vi "Error Cluster From Error Code_subroutine.vi"(4 "is warning? (False)":bool, 5 "show call chain? (False)":bool, 6 "error in (no error)":errorcluster, 8 "error message (\"\")":string, 9 "error code (0)":i32) -> (0 "error out":errorcluster)   [LabVIEW 2019, in "Tools.lvlib"]
doc: "Converts an error or warning code to an error cluster. This VI is useful when you receive a return value from a shared library call or when you return user-defined error codes."
uses:
  <vilib>/Utility/error.llb/whitespace.ctl
  Tools.lvlib
panel:
  in  "call chain header":string="\n<b>Complete call chain:</b>"
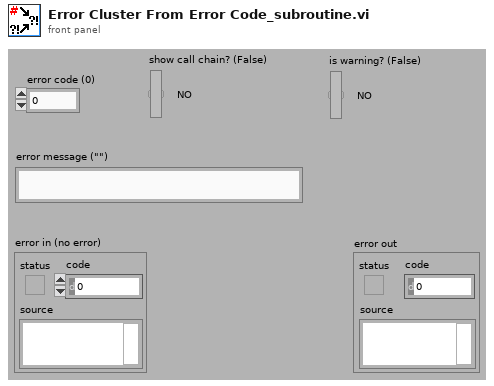
[diagram p1: front panel]
types:
  T1 = typedef "whitespace.ctl" = u16
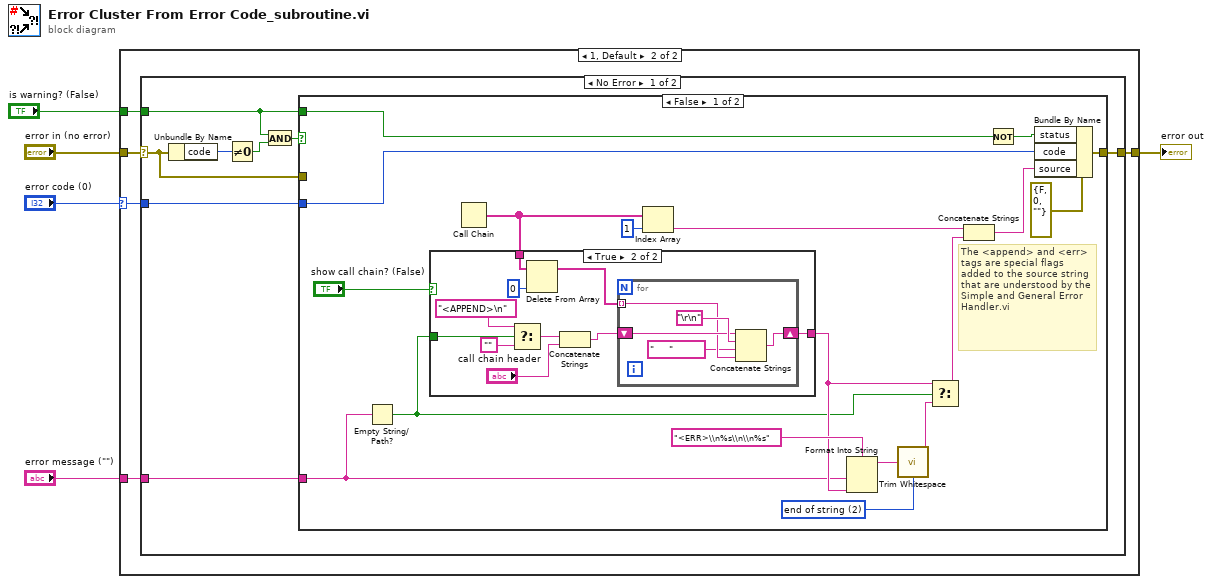
[diagram p0: block diagram]
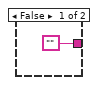
[diagram p3: hidden frame]
diagram:
  n1 = case shown="1, Default" "error code (0)" {
    selector: "error code (0)" -> [_ w9]
    tunnel: [w6 w11] -> w5
    tunnel: "error in (no error)" -> [w6 w10]
    tunnel: "error message (\"\")" -> [_ w8]
    tunnel: "is warning? (False)" -> [_ w7]
    frame 0 {
      # "If the error code in equals zero, then propagate the error in cluster regardless of its value."
    }
    frame 1, Default {
      n2 = case shown="No Error" w10 {
        selector: w10 -> [w14 w55]
        tunnel: [w19 w55] -> w11
        tunnel: w9 -> [w18 _]
        tunnel: w8 -> [w13 _]
        tunnel: w7 -> [w12 _]
        frame No Error {
          n3 = Unbundle By Name(w14) -> ("code"=w17:i32)
          n4 = Not Equal To 0?(x=w17) -> (x != 0?=w15:bool)
          n5 = And(x=w12, y=w15) -> (x .and. y?=w16:bool)
          n6 = case shown="False" w16 {
            tunnel: [w37 w54] -> w19
            tunnel: w18 -> [w33 _]
            tunnel: w14 -> [_ w54]
            tunnel: w12 -> [w30 _]
            tunnel: w13 -> [w25 _]
            frame False {
              w21 = T1 2 items=["both", "start of string", "end of string"] ("location (both)")
              # "The <append> and <err> tags are special flags added to the source string that are understood by the Simple and General Error Handler.vi"
              n7 = Empty String/Path?(string/path=w25) -> (empty?=w24:bool)
              n8 = Call Chain() -> (call chain=w31:string[])
              n9 = case shown="True" "show call chain? (False)" {
                tunnel: ["" w48] -> w27
                tunnel: w31 -> [_ w46]
                tunnel: w24 -> [_ w42]
                frame False {
                }
                frame True {
                  n10 = Select(t="<APPEND>\n", s=w42, f="") -> (s? t:f=w39:string)
                  n11 = Delete From Array(array=w46, index=0) -> (array with subset deleted=w45:string[])  [unwired: 1 in, 1 out]
                  n12 = Concatenate Strings(w39, "call chain header") -> (w43:string)
                  n13 = for {
                    tunnel: w45 -> [w50] mode=indexing
                    shift-right: [w53] -> w48
                    shift-left: w43 -> [w51]
                    n14 = Concatenate Strings(w51, "\r\n", "     ", w50) -> (w53:string)
                  }
                }
              }
              n15 = Index Array(array=w31, index=1) -> (element=w20:string)
              n16 = Format Into String(format string="<ERR>\\n%s\\n\\n%s", w25, w27) -> (resulting string=w23:string)  [unwired: 2 in, 1 out]
              n17 = call <vilib>:"Trim Whitespace.vi"("string"=w23, "location (both)"=w21) -> ("trimmed string"=w22:string)
              n18 = Select(t=w27, s=w24, f=w22) -> (s? t:f=w26:string)
              n19 = Concatenate Strings(w20, w26) -> (w35:string)
              n20 = Not(x=w30) -> (.not. x?=w34:bool)
              n21 = Bundle By Name(cluster=errorcluster {"status"=FALSE, "code"=0, "source"=""} ("error out"), "status"=w34, "code"=w33, "source"=w35) -> (w37:errorcluster)
            }
            frame True {
              # "If the error code input is setting a warning, and a warning is already set on the wire, then we\ngo with the one already on the wire."
            }
          }
        }
        frame Error {
          # "An error in trumps any error code input."
        }
      }
    }
  }
  "error out" <- w5
